vi "State_Machine.vi"(8 "error in (no error)":errorcluster caption="entrée d'erreur (pas d'erreur)", 11 "Get_Voltage en entrée":refnum<class "P2056_Set_DeviceID.lvclass">) -> (0 "error out":errorcluster caption="sortie d'erreur", 2 "Json_String":string, 3 "Get_Voltage en sortie":refnum<class "P2056_Set_DeviceID.lvclass">)   [LabVIEW 2020, in "Library Test.lvlib" / "P2056_Set_DeviceID.lvclass"]
uses:
  P2056_Set_DeviceID.lvclass
  C:/Users/ngarcin/OneDrive - Altyor/Standard TB/Suite TB45/Class/Test/P2056_Send_Command_UART/P2056_Send_Command_UART.lvclass
  Commun VI/TypeDef/Variable Printable.ctl
  P2056_Send_Command_UART.lvclass
  Commun VI/Library Commun.lvlib
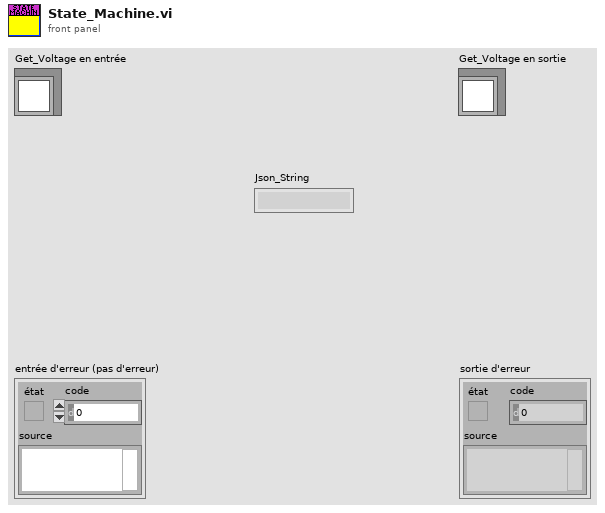
[diagram p1: front panel]
types:
  T1 = typedef "Variable Printable.ctl" = string
  T2 = enum16{"Get Variable", "Get All Variables", "Set Variable", "Delete Variable", "Delete All Variable"}
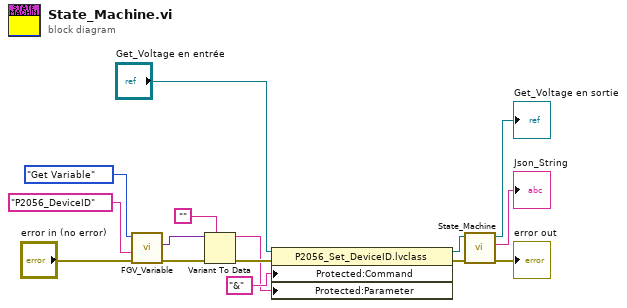
[diagram p0: block diagram]
diagram:
  n1 = call "FGV_Variable.vi"("error in (no error)"="error in (no error)", "Variable"=T1 "P2056_DeviceID", "Function"=T2."Get Variable") -> ("error out"=w6:errorcluster, "Data Out"=w4:variant)  [unwired: 6 in, 1 out]
  n2 = Variant To Data(error in=w6, type="", Variant=w4) -> (data=w2:string, error out=w5:errorcluster)
  n3 = property class="P2056_Set_DeviceID.lvclass"(reference="Get_Voltage en entrée", error in=w5, "Protected:Command"="&" ("chaîne"), "Protected:Parameter"=w2) -> (reference out=w13:refnum<class "P2056_Set_DeviceID.lvclass">, error out=w12:errorcluster)
  n4 = call-parent "State_Machine.vi"("error in (no error)"=w12, "Get_Voltage en entrée"=w13) -> ("error out"=→"error out":errorcluster, "Json_String"=→"Json_String":string, "Get_Voltage en sortie"=→"Get_Voltage en sortie":refnum<class "P2056_Set_DeviceID.lvclass">)  [unwired: 7 in]
